vi "BarrettReduction.vi"(1 "mu":cluster{"Boolean":bool, "Array":u64[]}, 2 "b":cluster{"Boolean":bool, "Array":u64[]}, 3 "a":cluster{"Boolean":bool, "Array":u64[]}) -> (0 "a % b":cluster{"Boolean":bool, "Array":u64[]})   [LabVIEW 2023]
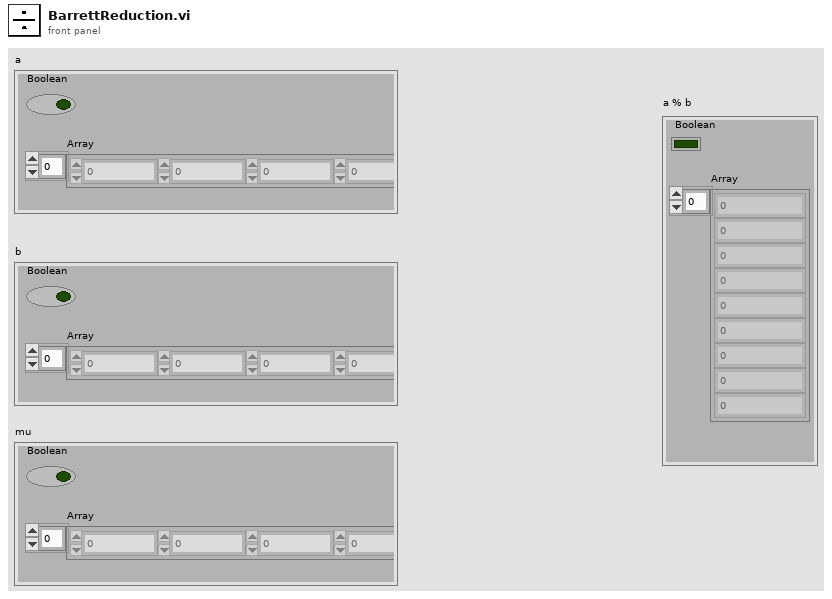
[diagram p1: front panel]
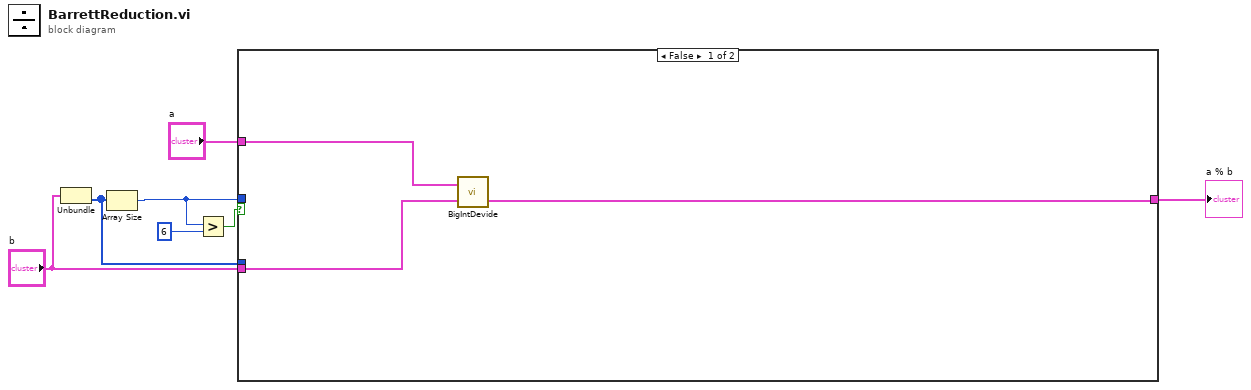
[diagram p0: block diagram]
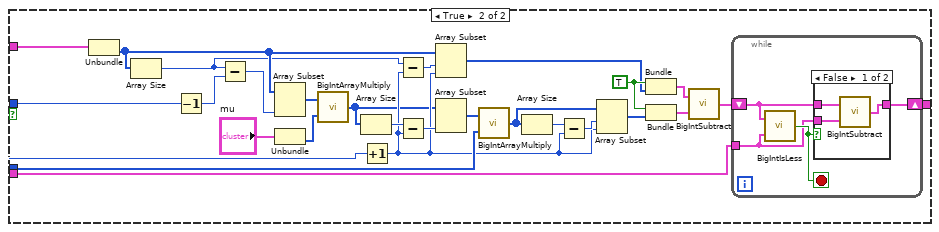
[diagram p2: hidden frame]
diagram:
  n1 = Unbundle("b") -> ("Array"=w7:u64[])  [unwired: 1 out]
  n2 = Array Size(array=w7) -> (size(s)=w3:i32)
  n3 = Greater?(x=w3, y=6) -> (0:w2:bool)
  n4 = case shown="False" w2 {
    tunnel: w7 -> [_ w29]
    tunnel: "b" -> [w9 w19]
    tunnel: [w8 w14] -> w5
    tunnel: w3 -> [_ w12]
    tunnel: "a" -> [w10 w11]
    frame False {
      n5 = call "BigIntDevide.vi"("b"=w9, "a"=w10) -> ("a % b"=w8:cluster{"Boolean":bool, "Array":u64[]})  [unwired: 1 out]
    }
    frame True {
      w24 = TRUE
      n6 = Unbundle(w11) -> ("Array"=w32:u64[])  [unwired: 1 out]
      n7 = Array Size(array=w32) -> (size(s)=w13:i32)
      n8 = Decrement(x=w12) -> (x-1=w37:i32)
      n9 = Subtract(x=w13, y=w37) -> (x-y=w36:i32)
      n10 = Array Subset(array=w32, length=w36) -> (w30:u64[])  [unwired: 1 in]
      n11 = Unbundle("mu") -> ("Array"=w17:u64[])  [unwired: 1 out]
      n12 = call "BigIntArrayMultiply.vi"("b"=w17, "a"=w30) -> ("a * b"=w16:u64[])
      n13 = Array Size(array=w16) -> (size(s)=w34:i32)
      n14 = Increment(x=w12) -> (x+1=w25:i32)
      n15 = Subtract(x=w13, y=w25) -> (x-y=w31:i32)
      n16 = Subtract(x=w34, y=w25) -> (x-y=w33:i32)
      n17 = Array Subset(array=w32, index=w31, length=w25) -> (w23:u64[])
      n18 = Array Subset(array=w16, length=w33) -> (w15:u64[])  [unwired: 1 in]
      n19 = call "BigIntArrayMultiply.vi"("b"=w29, "a"=w15) -> ("a * b"=w28:u64[])
      n20 = Array Size(array=w28) -> (size(s)=w27:i32)
      n21 = Subtract(x=w27, y=w25) -> (x-y=w26:i32)
      n22 = Array Subset(array=w28, index=w26, length=w25) -> (w22:u64[])
      n23 = Bundle(w24, w23) -> (w21:cluster{bool, u64[]})  [unwired: 1 in]
      n24 = Bundle(w24, w22) -> (w20:cluster{bool, u64[]})  [unwired: 1 in]
      n25 = call "BigIntSubtract.vi"("b"=w20, "a"=w21) -> ("a - b"=w18:cluster{"Boolean":bool, "Array":u64[]})
      n26 = while {
        tunnel: w19 -> [w39]
        shift-right: [w38] -> w14
        shift-left: w18 -> [w40]
        stop <- w41 stop-if-true
        n27 = call "BigIntIsLess.vi"("b"=w39, "a"=w40) -> ("a < b"=w41:bool)
        n28 = case shown="False" w41 {
          tunnel: [w42 w45] -> w38
          tunnel: w40 -> [w44 w45]
          tunnel: w39 -> [w43 _]
          frame False {
            n29 = call "BigIntSubtract.vi"("b"=w43, "a"=w44) -> ("a - b"=w42:cluster{"Boolean":bool, "Array":u64[]})
          }
          frame True {
          }
        }
      }
    }
  }
  "a % b" <- w5
